vi "Speed Control 4.vi"(11 "queue in":refnum<queue>) -> ()   [LabVIEW 2014]
uses:
  controls/UI Data.ctl
  controls/Control ConfigurationSam.ctl
  controls/EncoderController.ctl
  <vilib>/Platform/TimedLoop/XDataNode/timing_clust.ctl
  <vilib>/Platform/TimedLoop/XDataNode/nitl_modes.ctl
  <vilib>/Platform/TimedLoop/XDataNode/wakeup.ctl
  controls/Control StateSam.ctl
  <vilib>/myRIO/Instrument Drivers/Onboard IO/PWM/typedefs/PWM Reference.ctl
  <vilib>/myRIO/Common/Instrument Driver Framework/Utilities/typedefs/myRIO Generic Hardware Reference.ctl
  <vilib>/myRIO/Common/Instrument Driver Framework/Utilities/typedefs/Hardware Version Enum.ctl
  <vilib>/myRIO/Common/Instrument Driver Framework/Utilities/typedefs/myRIO v1.0 Reference.ctl
  <vilib>/myRIO/Common/Instrument Driver Framework/Utilities/typedefs/Generic FPGA Reference.ctl
  <vilib>/myRIO/Common/Instrument Driver Framework/myRIO v1.0/PWM/typedefs/PWM Channels Enum.ctl
  <vilib>/myRIO/Instrument Drivers/Onboard IO/PWM/typedefs/PWM Configuration.ctl
  <vilib>/userdefined/High Color/nirio_resource_hc.ctl
  <vilib>/myRIO/Common/Instrument Driver Framework/Utilities/vis/Is FPGA Ref Available.vi
  <vilib>/myRIO/Common/Instrument Driver Framework/myRIO v1.0/PWM/vis/myRIO v1.1 Open PWM.vi
  <vilib>/myRIO/Instrument Drivers/Onboard IO/PWM/vis/Set Duty Cycle and Frequency.vi
  <vilib>/myRIO/Common/Instrument Driver Framework/Utilities/vis/Validate Channels.vi
  <vilib>/myRIO/Common/Instrument Driver Framework/myRIO v1.0/PWM/vis/myRIO v1.0 Reserve PWM.vi
  <vilib>/myRIO/Common/Instrument Driver Framework/myRIO v1.0/PWM/vis/myRIO v1.0 Build MUX Configuration PWM.vi
  <vilib>/myRIO/Common/Instrument Driver Framework/myRIO v1.0/Resource Manager/vis/myRIO v1.0 Reserve Channel List.vi
  <vilib>/myRIO/Common/Instrument Driver Framework/myRIO v1.0/Resource Manager/vis/myRIO v1.0 Create Configuration List.vi
  <vilib>/myRIO/Common/Instrument Driver Framework/myRIO v1.0/Resource Manager/vis/myRIO v1.0 Reserve Channel.vi
  <vilib>/myRIO/Common/Instrument Driver Framework/myRIO v1.0/Resource Manager/vis/myRIO v1.0 Unreserve Channel.vi
  <vilib>/myRIO/Common/Instrument Driver Framework/myRIO v1.0/Resource Manager/vis/myRIO v1.0 Build Mutex Name.vi
  <vilib>/Utility/VariantDataType/GetNumericInfo.vi
  <vilib>/Utility/error.llb/Error Cluster From Error Code.vi
  <vilib>/myRIO/Common/Instrument Driver Framework/myRIO v1.0/myRIO v1.1 Open.vi
  <vilib>/myRIO/Common/Instrument Driver Framework/Utilities/vis/IO Manager.vi
  <vilib>/myRIO/Common/Instrument Driver Framework/Utilities/vis/Configuration Manager.vi
  <vilib>/myRIO/Common/Instrument Driver Framework/myRIO v1.0/Resource Manager/vis/myRIO v1.0 Configure IO.vi
  <vilib>/myRIO/Common/Instrument Driver Framework/myRIO v1.0/myRIO v1.0 Close.vi
  <vilib>/myRIO/Common/Instrument Driver Framework/myRIO v1.0/PWM/vis/myRIO v1.0 Write PWM.vi
  <vilib>/addons/control/pid/pid.llb/PID (DBL Array).vi
  <vilib>/addons/control/pid/pid.llb/PID Percentage to EGU (DBL Array).vi
  <vilib>/myRIO/Express VI/Onboard IO/PWM/PWM Express VI.xnode
  <vilib>/myRIO/Instrument Drivers/Onboard IO/PWM/vis/myRIO PWM Open.xnode
  <vilib>/platform/TimedLoop/XDataNode/XDataNode.xnode
  <vilib>/addons/control/pid/NI_PID_pid.lvlib
  <vilib>/Platform/TimedLoop/XDataNode/XDNodeRunTimeDep.lvlib
  <vilib>/myRIO/Instrument Drivers/Onboard IO/PWM/PWM.lvlib
panel:
  out "Motor1Output":dbl
  out "Velocity1 RPM":dbl
  out "Motor4Output":dbl
  out "Velocity4 RPM":dbl
  # "0.8, 0. 0 is stable but theres a large offset\nsystem is slow to settle, increase Ti"
  # "Kp=2.04, Ti=0.15, Td=0.0375"
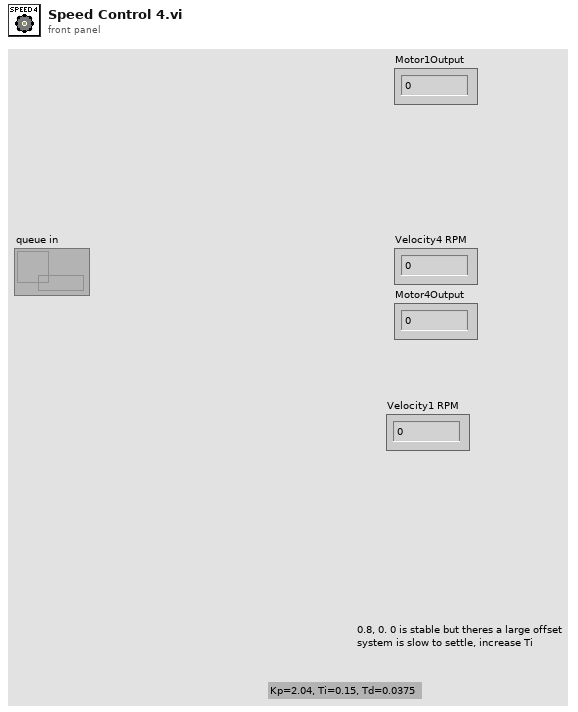
[diagram p1: front panel]
types:
  T1 = typedef "Control ConfigurationSam.ctl" = cluster{"PID Gains":cluster{"proportional gain (Kc)":dbl, "integral gain (Kc*Ts/Ti)":dbl, "derivative gain (Kc*Td/Ts)":dbl}, "Output Range":cluster{"output high":dbl, "output low":dbl}}
  T2 = cluster{bool, "Tick Count(uSec)":u32, "Counter Value":i32, "x-y":i32}
  T3 = cluster{"proportional gain (Kc)":dbl, "integral gain (Kc*Ts/Ti)":dbl, "derivative gain (Kc*Td/Ts)":dbl}
  T4 = cluster{"proportional gain (Kc)":dbl, "integral gain (Kc*Ts/Ti)":dbl, "derivative gain (Kc*Td/Ts)":dbl}[]
  T5 = typedef "XDNodeRunTimeDep.lvlib/timing_clust.ctl" = cluster{"Expected End [f-1]":u64, "Actual End [f-1]":u64, "Finished Late? [f-1]":bool, "Expected End [i-1]":u64, "Actual End [i-1]":u64, "Finished Late? [i-1]":bool, "Expected Start [i]":u64, "Actual Start [i]":u64, "Expected Start [f]":u64, "Actual Start [f]":u64, "Source Name":string, "Structure Name":string, "Period":i64, "Deadline":i64, "Offset":i64, "Start":i64, "Priority":i32, "Timeout":i32, "Mode":T6, "Wakeup Reason":T7, "Error":errorcluster, "Source Type":string, "Secondary Source Type":string, "Global End Time":u64, "Global Start Time":u64, "Frame Duration":u64, "Iteration Duration":u64, "Assigned CPU":i32, "I/O Scan Engine Mode":u32}
  T6 = typedef "XDNodeRunTimeDep.lvlib/nitl_modes.ctl" = enum32{"No Change", "Process missed periods, maintain original phase", "Discard missed periods, maintain original phase", "Process missed periods, ignore original phase", "Discard missed periods, ignore original phase"}
  T7 = typedef "XDNodeRunTimeDep.lvlib/wakeup.ctl" = enum32{"Normal", "Aborted", "Asynchronous wakeup", "Timing source error", "Timed loop error", "Timeout"}
  T8 = typedef "PWM.lvlib/PWM Reference.ctl" = cluster{"myRIO Reference":T9, "PWM Channels Enum":T13, "PWM Configuration":T14}
  T9 = typedef "myRIO Generic Hardware Reference.ctl" = cluster{"myRIO Model":T10, "myRIO Hardware Reference":T11}
  T10 = typedef "Hardware Version Enum.ctl" = enum16{"Unknown", "myRIO-1900", "myRIO-1950"}
  T11 = typedef "myRIO v1.0 Reference.ctl" = cluster{"Generic FPGA Reference":T12, "Allow multiple opens":bool}
  T12 = typedef "Generic FPGA Reference.ctl" = refnum<k20>
  T13 = typedef "PWM Channels Enum.ctl" = enum16{"Not Connected", "C/PWM0", "C/PWM1", "A/PWM0", "A/PWM1", "A/PWM2", "B/PWM0", "B/PWM1", "B/PWM2"}
  T14 = typedef "PWM.lvlib/PWM Configuration.ctl" = cluster{"Frequency":dbl, "Duty Cycle":dbl}
  T15 = typedef "nirio_resource_hc.ctl" = tag
  T16 = typedef "EncoderController.ctl" = cluster{"Sample time (uS)":u32, "Reset":bool}
  T17 = typedef "EncoderIndicator.ctl" = cluster{"Position":dbl, "Velocity RPM":dbl, "Velocity RPS":dbl}
  T18 = typedef "Control StateSam.ctl" = enum16{"", "Control State (PID)", "Safe State"}
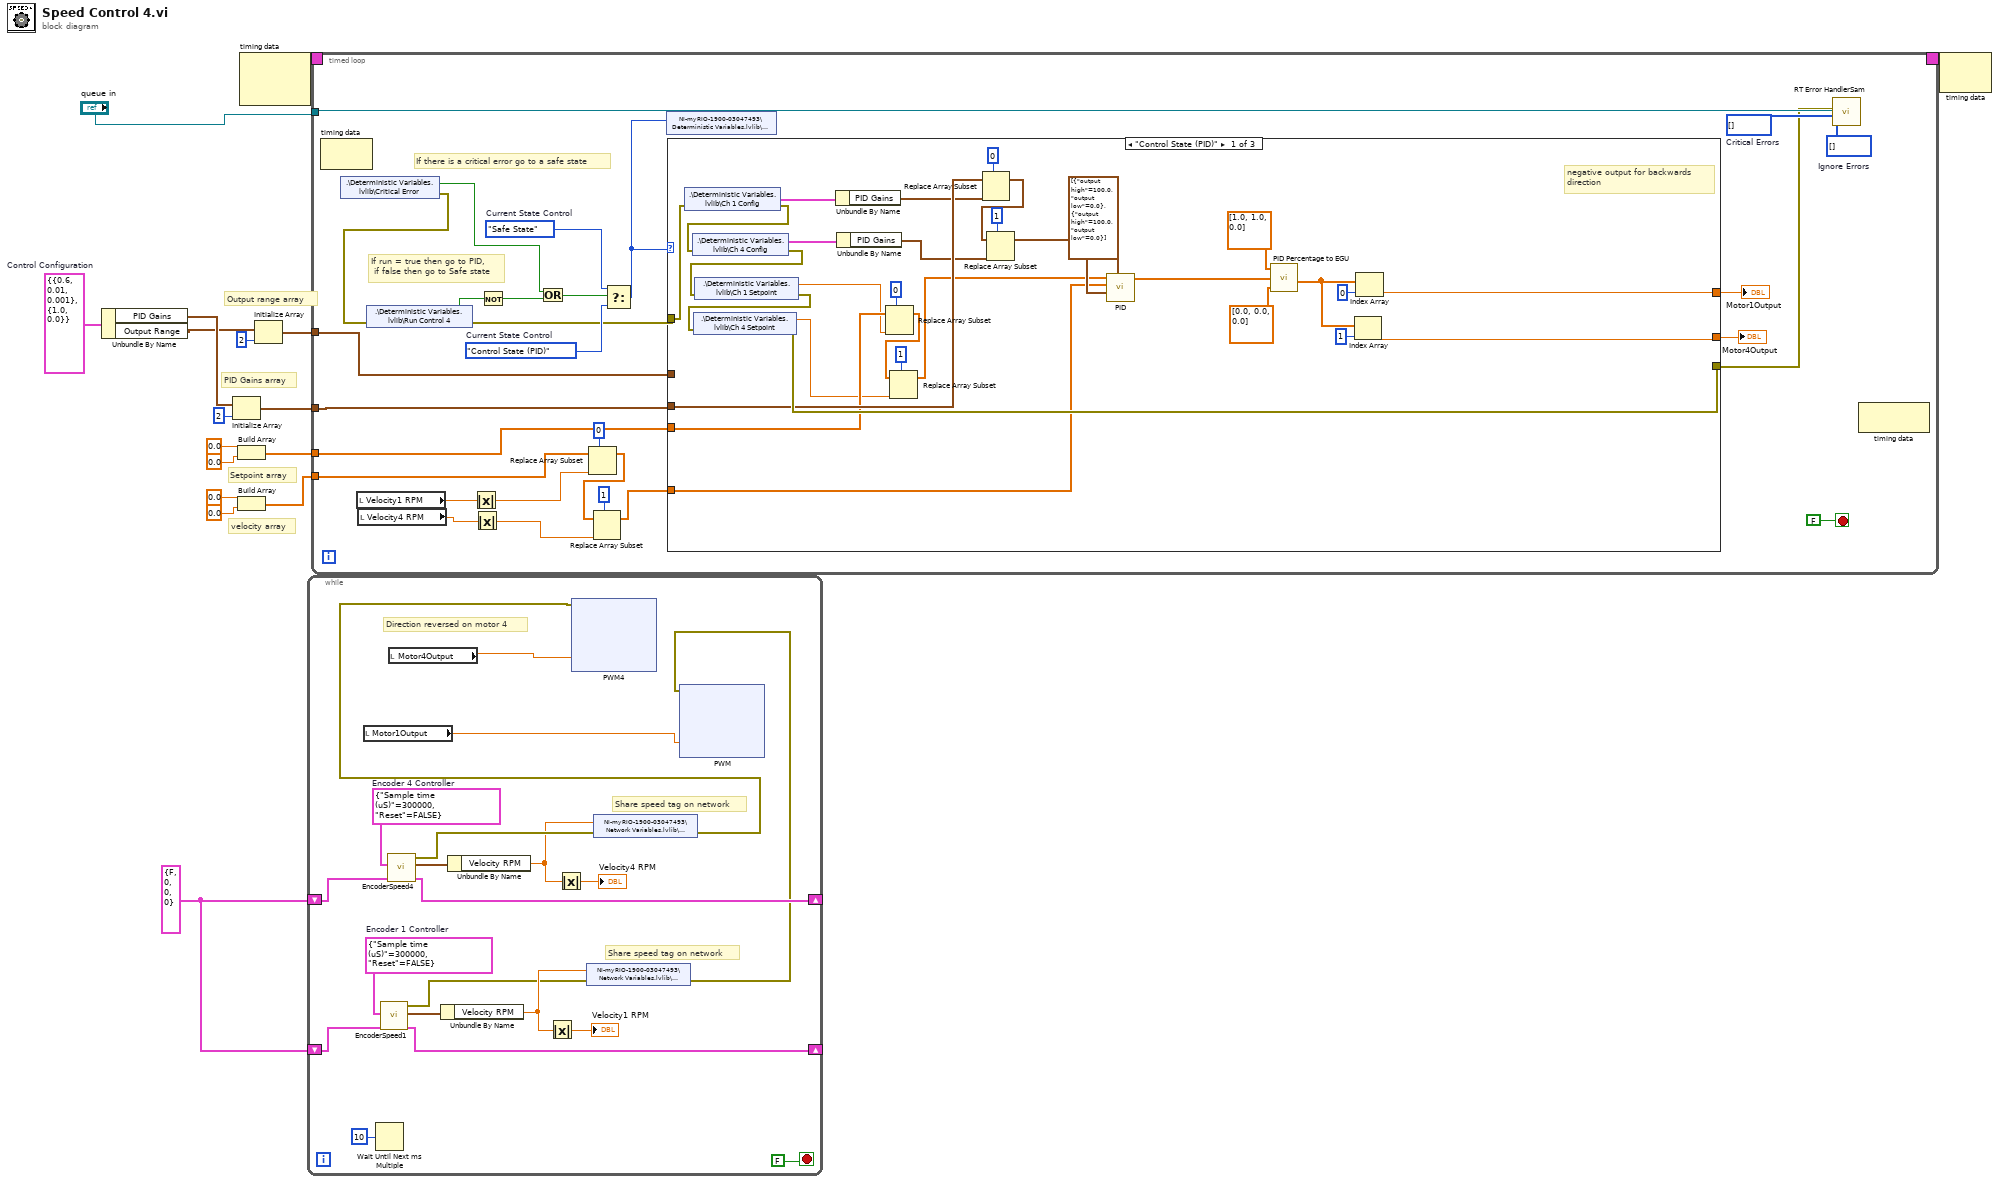
[diagram p0: block diagram]
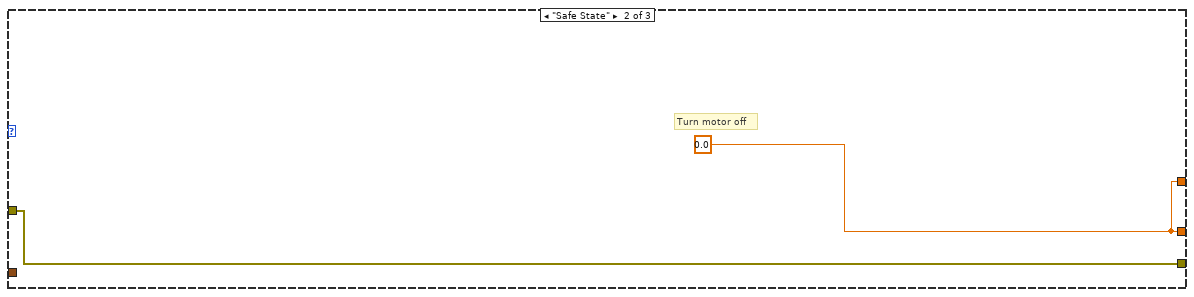
[diagram p2: hidden frame]
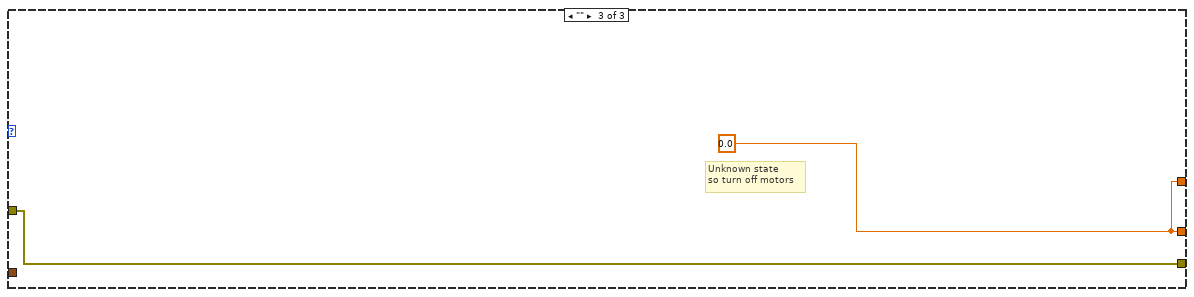
[diagram p3: hidden frame]
diagram:
  w5 = T1 {"PID Gains"={"proportional gain (Kc)"=0.6, "integral gain (Kc*Ts/Ti)"=0.01, "derivative gain (Kc*Td/Ts)"=0.001}, "Output Range"={"output high"=1.0, "output low"=0.0}}  # Control Configuration
  w14 = T2 {FALSE, "Tick Count(uSec)"=0, "Counter Value"=0, "x-y"=0} ("Cluster out")
  # "Output range array"
  # "velocity array"
  # "PID Gains array"
  # "Setpoint array"
  n1 = Unbundle By Name(w5) -> ("PID Gains"=w4:T3, "Output Range"=w2:cluster{"output high":dbl, "output low":dbl})
  n2 = Initialize Array(w4, 2 ("dimension size")) -> (w12:T4)
  n3 = Build Array(0.0, 0.0) -> (w9:dbl[])
  n4 = Build Array(0.0, 0.0) -> (w6:dbl[])
  n5 = node-c288() -> (w17:T5)  [unwired: 2 in]
  n6 = Initialize Array(w2, 2 ("dimension size")) -> (w1:cluster{"output high":dbl, "output low":dbl}[])
  n7 = while {
    shift-right: [w33] -> _
    shift-left: w14 -> [w34]
    shift-right: [w23] -> _
    shift-left: w14 -> [w22]
    stop <- FALSE stop-if-true
    w24 = T16 {"Sample time (uS)"=300000, "Reset"=FALSE}  # Encoder 1 Controller
    w37 = T16 {"Sample time (uS)"=300000, "Reset"=FALSE}  # Encoder 4 Controller
    # "Direction reversed on motor 4"
    # "Share speed tag on network"
    # "Share speed tag on network"
    n8 = local read "Motor1Output"() -> (w21:dbl)
    n9 = Wait Until Next ms Multiple(millisecond multiple=u32 10) -> ()  [unwired: 1 out]
    n10 = call "EncoderSpeed1.vi"("Cluster in"=w22, "Encoder 1 Controller"=w24) -> ("Cluster out"=w23:T2, "Encoder 1 Indicator"=w25:T17, "error out"=w26:errorcluster)  [unwired: 7 in]
    n11 = call "EncoderSpeed4.vi"("Cluster in"=w34, "Encoder 4 Controller"=w37) -> ("Cluster out"=w33:T2, "Encoder 4 Indicator"=w36:T17, "error out"=w35:errorcluster)  [unwired: 7 in]
    n12 = local read "Motor4Output"() -> (w18:dbl)
    n13 = Unbundle By Name(w25) -> ("Velocity RPM"=w28:dbl)
    n14 = Unbundle By Name(w36) -> ("Velocity RPM"=w29:dbl)
    n15 = Absolute Value(x=w28) -> (abs(x)=→"Velocity1 RPM":dbl)
    n16 = Absolute Value(x=w29) -> (abs(x)=→"Velocity4 RPM":dbl)
    n17 = shared-variable "NI-myRIO-1900-03047493\\Network Variables.lvlib\\SpeedMotor1"(w28, error in=w26) -> (error out=w19:errorcluster)
    n18 = shared-variable "NI-myRIO-1900-03047493\\Network Variables.lvlib\\SpeedMotor4"(w29, error in=w35) -> (error out=w20:errorcluster)
    n19 = xnode "PWM4"("Duty Cycle"=w18, "error in (no error)"=w20) -> ()  [unwired: 1 out]
    n20 = xnode "PWM"("Duty Cycle"=w21, "error in (no error)"=w19) -> ()  [unwired: 1 out]
  }
  n21 = timed-loop {
    timing: w17 -> [_]
    timing-out: [_] -> w16
    tunnel: "queue in" -> [w123]
    tunnel: w12 -> [w120]
    tunnel: w9 -> [w119]
    tunnel: w6 -> [w112]
    tunnel: w1 -> [w118]
    stop <- FALSE stop-if-true
    w124 = i32[] []  # Critical Errors
    w125 = i32[] []  # Ignore Errors
    w132 = Control_StateSam."Control State (PID)"  # Current State Control
    w133 = Control_StateSam."Safe State"  # Current State Control
    # "If there is a critical error go to a safe state"
    # "If run = true then go to PID,\n if false then go to Safe state"
    n22 = node-c288() -> ()  [unwired: 1 in, 1 out]
    n23 = shared-variable ".\\Deterministic Variables.lvlib\\Critical Error"() -> (w129:bool, error out=w127:errorcluster)  [unwired: 1 in]
    n24 = local read "Velocity1 RPM"() -> (w116:dbl)
    n25 = local read "Velocity4 RPM"() -> (w115:dbl)
    n26 = shared-variable ".\\Deterministic Variables.lvlib\\Run Control 4"(error in=w127) -> (w134:bool, error out=w126:errorcluster)
    n27 = Absolute Value(x=w116) -> (abs(x)=w108:dbl)
    n28 = Absolute Value(x=w115) -> (abs(x)=w109:dbl)
    n29 = Not(x=w134) -> (.not. x?=w130:bool)
    n30 = Or(x=w129, y=w130) -> (x .or. y?=w128:bool)
    n31 = Replace Array Subset(array=w112, new element=w108, index=0) -> (w111:dbl[])
    n32 = Replace Array Subset(array=w111, new element=w109, index=1) -> (w110:dbl[])
    n33 = Select(t=w133, s=w128, f=w132) -> (s? t:f=w131:T18)
    n34 = shared-variable "NI-myRIO-1900-03047493\\Deterministic Variables.lvlib\\Control State 4"(w131) -> ()  [unwired: 1 in, 1 out]
    n35 = case shown="\"Control State (PID)\"" w131 {
      tunnel: [w145 w167 w169] -> w122
      tunnel: w126 -> [w166 w168 w170]
      tunnel: [w161 w168 w170] -> w121
      tunnel: w120 -> [w157 _ _]
      tunnel: w119 -> [w141 _ _]
      tunnel: w118 -> [_ _ _]
      tunnel: [w146 w167 w169] -> w117
      tunnel: w110 -> [w144 _ _]
      frame "Control State (PID)" {
        # "negative output for backwards \ndirection"
        n36 = shared-variable ".\\Deterministic Variables.lvlib\\Ch 1 Config"(error in=w166) -> (w154:T1, error out=w164:errorcluster)
        n37 = shared-variable ".\\Deterministic Variables.lvlib\\Ch 4 Config"(error in=w164) -> (w165:T1, error out=w163:errorcluster)
        n38 = shared-variable ".\\Deterministic Variables.lvlib\\Ch 1 Setpoint"(error in=w163) -> (w140:dbl, error out=w162:errorcluster)
        n39 = shared-variable ".\\Deterministic Variables.lvlib\\Ch 4 Setpoint"(error in=w162) -> (w139:dbl, error out=w161:errorcluster)
        n40 = Unbundle By Name(w154) -> ("PID Gains"=w156:T3)
        n41 = Unbundle By Name(w165) -> ("PID Gains"=w155:T3)
        n42 = Replace Array Subset(array=w141, new element=w140, index=0) -> (w138:dbl[])
        n43 = Replace Array Subset(array=w138, new element=w139, index=1) -> (w137:dbl[])
        n44 = Replace Array Subset(array=w157, new element=w156, index=0) -> (w158:T4)
        n45 = Replace Array Subset(array=w158, new element=w155, index=1) -> (w153:T4)
        n46 = call-poly <vilib>:"PID.vi"("output range"=cluster{"output high":dbl, "output low":dbl}[] [{"output high"=100.0, "output low"=0.0}, {"output high"=100.0, "output low"=0.0}], "PID gains"=w153, "process variable"=w144, "setpoint"=w137) -> ("output"=w152:dbl[])  [unwired: 6 in, 1 out]
        n47 = call-poly <vilib>:"PID Percentage to EGU.vi"("minimum (EGU)"=dbl[] [0.0, 0.0, 0.0] ("maximum (EGU)"), "% span"=w152, "maximum (EGU)"=dbl[] [1.0, 1.0, 0.0]) -> ("output (EGU)"=w147:dbl[])  [unwired: 1 in]
        n48 = Index Array(array=w147, index=1) -> (element=w145:dbl)
        n49 = Index Array(array=w147, index=0) -> (element=w146:dbl)
      }
      frame "Safe State" {
        w167 = 0.0 ("output (EGU)")
        # "Turn motor off"
      }
      frame "" {
        w169 = 0.0 ("output (EGU)")
        # "Unknown state\nso turn off motors"
      }
    }
    "Motor4Output" <- w122
    "Motor1Output" <- w117
    n50 = call "RT Error HandlerSam.vi"("Ignore Errors"=w125, "Critical Errors"=w124, "error to process"=w121, "queue in"=w123) -> ()  [unwired: 7 in, 1 out]
    n51 = node-c288() -> ()  [unwired: 1 in, 1 out]
  }
  n52 = node-c288(w16) -> ()  [unwired: 1 out]
